vi "background worker.vi"(11 "starburst in":refnum<class "starburst.lvclass">) -> ()   [LabVIEW 2015, in "starburst.lvclass"]
uses:
  starburst.lvclass
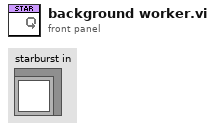
[diagram p1: front panel]
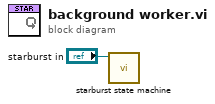
[diagram p0: block diagram]
diagram:
  n1 = call "starburst state machine.vi"("starburst in"="starburst in") -> ()  [unwired: 11 in]
